vi "FTW-Actor-InitializeBroker.vi"(0 "Uninitialized FTW Actor":refnum<class "FTW-Actor.lvclass">, 5 "Initialized Response":string, 11 "error in":errorcluster) -> (4 "FTW Actor":refnum<class "FTW-Actor.lvclass">, 6 "Incoming Messages":refnum<event-registration>, 15 "error out":errorcluster)   [LabVIEW 2013, in "FTW-Actor.lvclass"]
uses:
  FTW-Actor.lvclass
  Messaging/Message/FTW-Message.lvclass
  FTW-Actor.lvclass/FTW-Actor.ctl
  Context/Messaging/Broker/FTW-Actor-Broker.lvclass
panel:
  # "Inputs"
  # "Outputs"
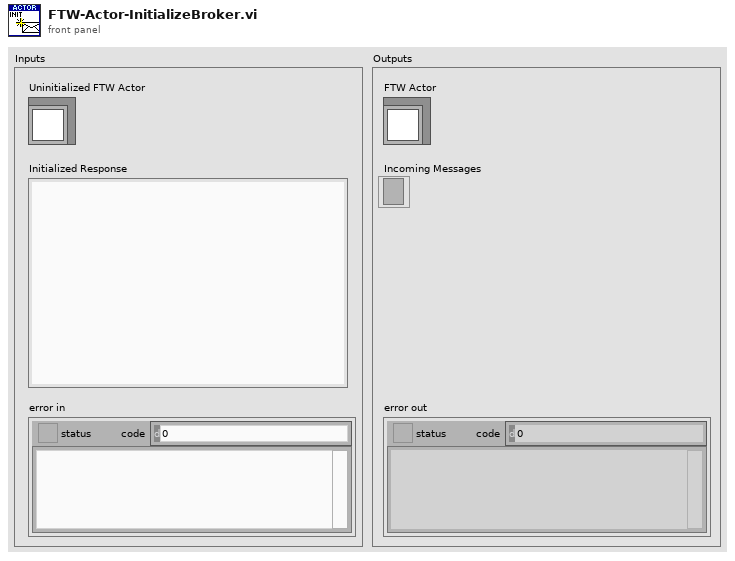
[diagram p1: front panel]
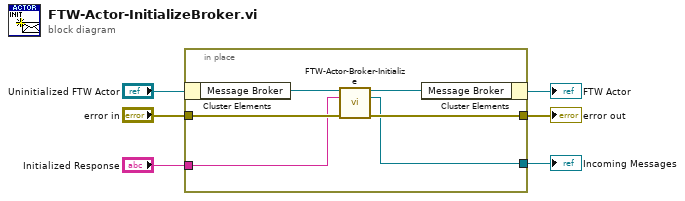
[diagram p0: block diagram]
diagram:
  n1 = in-place {
    in-place-border: "error in" -> [w8]
    in-place-border: [w10] -> w3
    in-place-border: [w9] -> w4
    in-place-border: "Initialized Response" -> [w7]
    n2 = in-place-cluster #1("Uninitialized FTW Actor") -> ("Message Broker"=w12:refnum<class "FTW-Actor-Broker.lvclass">)
    n3 = call "FTW-Actor-Broker-Initialize.vi"("FTW Message Broker"=w12, "Initialized Response"=w7, "error in"=w8) -> ("FTW Message Broker out"=w11:refnum<class "FTW-Actor-Broker.lvclass">, "Observer"=w9:refnum<event-registration>, "error out"=w10:errorcluster)  [unwired: 10 in]
    n4 = in-place-cluster #1("Message Broker"=w11) -> (→"FTW Actor":refnum<class "FTW-Actor.lvclass">)
  }
  "error out" <- w3
  "Incoming Messages" <- w4
